vi "移位寄存器2.vi"() -> ()   [LabVIEW 2023]
panel:
  out "循环结束以后输出":i32
  out "输出端寄存器 i":i32
  out "Numeric 2":i32
  out "Numeric":i32
  out "第三个输入寄存器 i-3":i32
  out "第二个输入寄存器 i-2":i32
  out "第一个输入寄存器  i-1":i32
  # "第一个例子要好好领会。 这东西真他妈。。。"
  # "移位寄存器2"
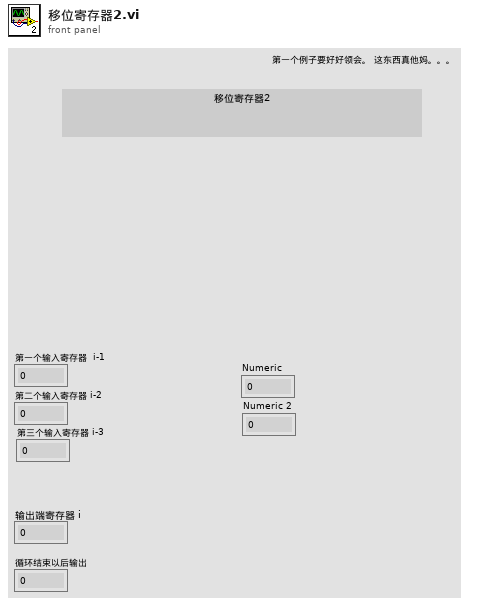
[diagram p1: front panel]
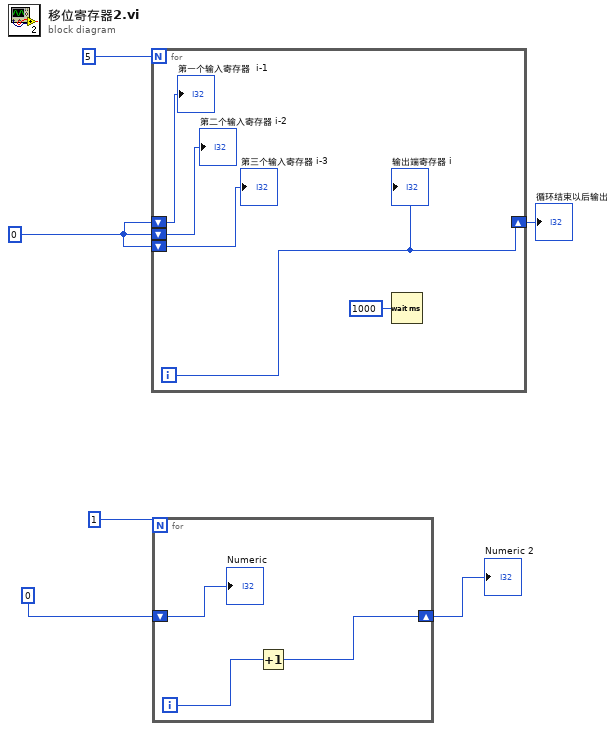
[diagram p0: block diagram]
diagram:
  w6 = 0
  n1 = for {
    N: 5 -> [_]
    shift-right: [w7] -> w1
    shift-left: w6 -> [w11]
    shift-left: w6 -> [w10]
    shift-left: w6 -> [w9]
    i -> [w7]
    n2 = Wait (ms)(milliseconds to wait=u32 1000) -> ()  [unwired: 1 out]
    "第一个输入寄存器  i-1" <- w11
    "第二个输入寄存器 i-2" <- w10
    "第三个输入寄存器 i-3" <- w9
    "输出端寄存器 i" <- w7
  }
  "循环结束以后输出" <- w1
  n3 = for {
    N: 1 -> [_]
    shift-right: [w13] -> w3
    shift-left: 0 -> [w12]
    i -> [w14]
    n4 = Increment(x=w14) -> (x+1=w13:i32)
    "Numeric" <- w12
  }
  "Numeric 2" <- w3
